vi "exercice5-1.vi"() -> ()   [LabVIEW 2013]
panel:
  out "Tableau":dbl[][](array[numeric])
  out "Angle":dbl[][](array[numeric])
  # "Cos"
  # "Tan"
  # "Sin"
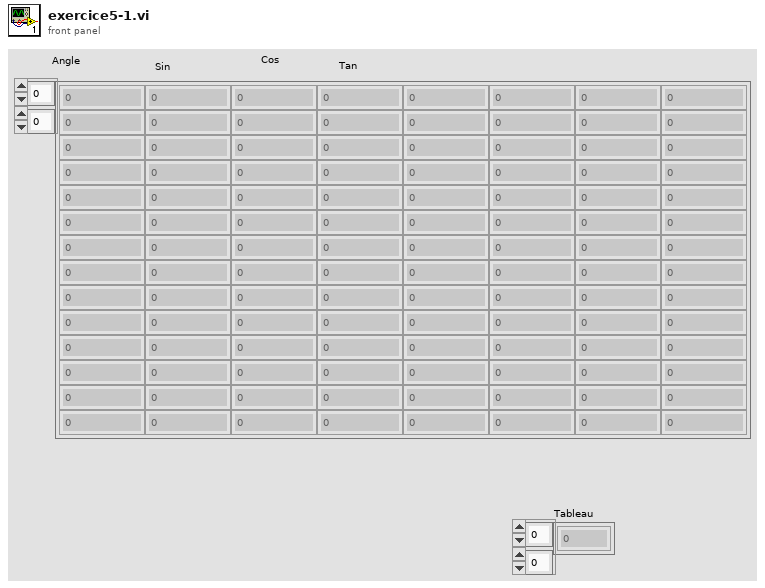
[diagram p1: front panel]
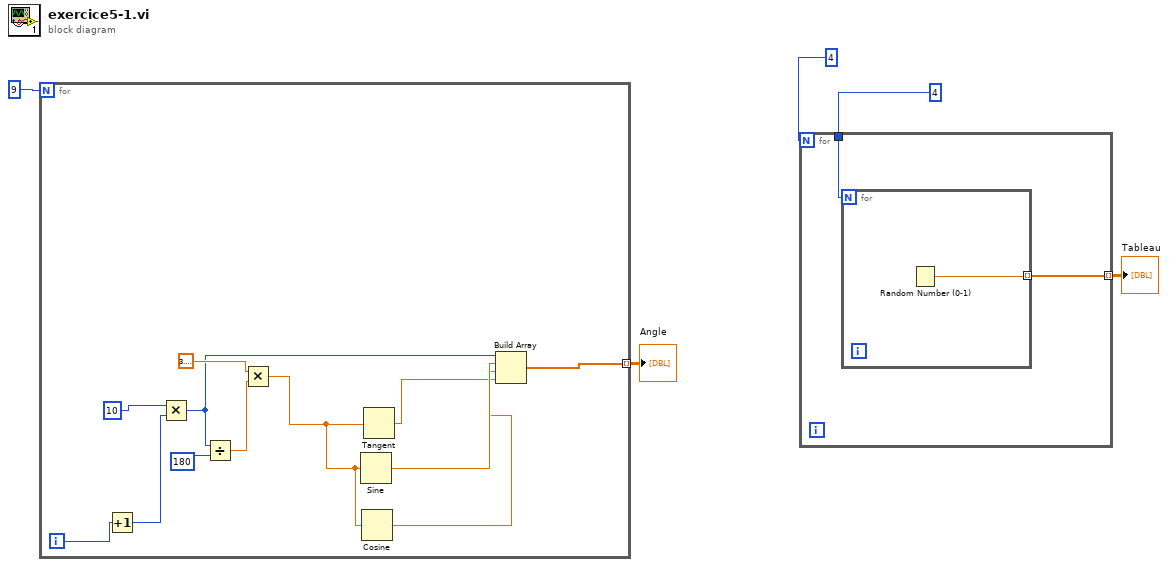
[diagram p0: block diagram]
diagram:
  n1 = for {
    N: 9 -> [_]
    tunnel: [w14] -> w4 mode=indexing
    i -> [w17]
    n2 = Increment(x=w17) -> (x+1=w16:i32)
    n3 = Multiply(x=10, y=w16) -> (x*y=w6:i32)
    n4 = Divide(x=w6, y=180) -> (x/y=w9:dbl)
    n5 = Multiply(x=3.141592653589793, y=w9) -> (x*y=w7:dbl)
    n6 = Sine(x=w7) -> (sin(x)=w13:dbl)
    n7 = Cosine(x=w7) -> (cos(x)=w12:dbl)
    n8 = Tangent(1:w7) -> (0:w11:dbl)
    n9 = Build Array(w6, w13, w12, w11) -> (w14:dbl[])
  }
  "Angle" <- w4
  n10 = for {
    N: 4 -> [_]
    tunnel: [w19] -> w3 mode=indexing
    tunnel: 4 -> [w18]
    n11 = for {
      N: w18 -> [_]
      tunnel: [w20] -> w19 mode=indexing
      n12 = Random Number (0-1)() -> (number: 0 to 1=w20:dbl)
    }
  }
  "Tableau" <- w3
